vi "Read Channel names.vi"(8 "error in (no error)":errorcluster, 11 "Channel Scanner Driver in":refnum<class "Channel Scanner Driver.lvclass">) -> (0 "error out":errorcluster, 2 "Channel names":string[](array[string]), 3 "Channel Scanner Driver out":refnum<class "Channel Scanner Driver.lvclass">)   [LabVIEW 2019, in "Channel Scanner Driver.lvclass"]
uses:
  Channel Scanner Driver.lvclass
  Channel Scanner Driver.lvclass/Channel Scanner Driver.ctl
  Read Scan Channels.vi
  Read Next channel idx.vi
  Simple VISA Reader/Simple VISA Reader Driver.lvclass
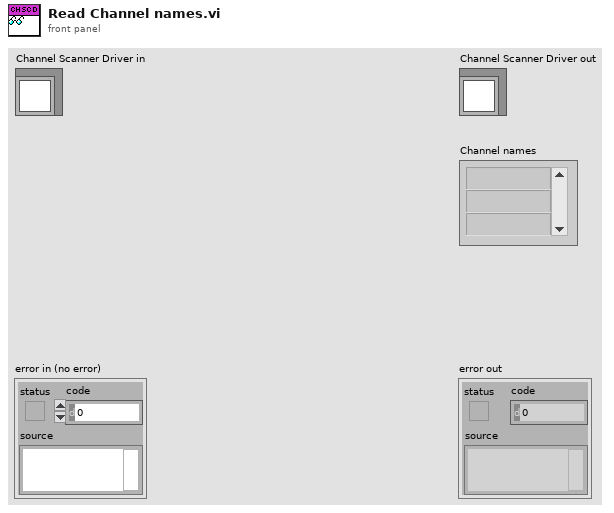
[diagram p1: front panel]
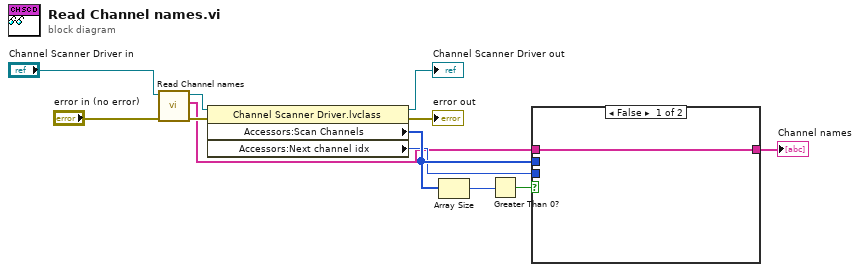
[diagram p0: block diagram]
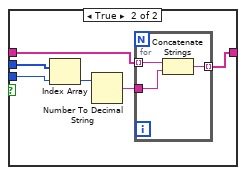
[diagram p2: hidden frame]
diagram:
  n1 = call-parent "Read Channel names.vi"("error in (no error)"="error in (no error)", "Instrument Driver in"="Channel Scanner Driver in") -> ("error out"=w12:errorcluster, "Channel names"=w3:string[], "Instrument Driver out"=w8:refnum<class "Channel Scanner Driver.lvclass">)  [unwired: 7 in]
  n2 = property class="Channel Scanner Driver.lvclass"(reference=w8, error in=w12) -> (reference out=→"Channel Scanner Driver out":refnum<class "Channel Scanner Driver.lvclass">, error out=→"error out":errorcluster, "Accessors:Scan Channels"=w5:i32[], "Accessors:Next channel idx"=w4:i32)
  n3 = Array Size(array=w5) -> (size(s)=w6:i32)
  n4 = Greater Than 0?(x=w6) -> (x > 0?=w2:bool)
  n5 = case shown="False" w2 {
    tunnel: w5 -> [_ w19]
    tunnel: w4 -> [_ w18]
    tunnel: w3 -> [w13 w17]
    tunnel: [w13 w14] -> w1
    frame False {
    }
    frame True {
      n6 = Index Array(array=w19, index=w18) -> (element=w16:i32)
      n7 = Number To Decimal String(number=w16) -> (decimal integer string=w15:string)  [unwired: 1 in]
      n8 = for {
        tunnel: w17 -> [w22] mode=indexing
        tunnel: w15 -> [w21]
        tunnel: [w20] -> w14 mode=indexing
        n9 = Concatenate Strings(w22, w21) -> (w20:string)
      }
    }
  }
  "Channel names" <- w1
